vi "PJT_13.vi"() -> ()   [LabVIEW 2019]
panel:
  out "매칭된 숫자":dbl
  out "반복횟수":i32
  in  "입력숫자":dbl
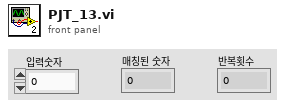
[diagram p1: front panel]
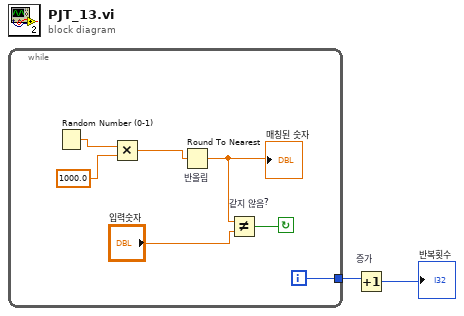
[diagram p0: block diagram]
diagram:
  n1 = while {
    tunnel: [w3] -> w2
    i -> [w3]
    stop <- w4 continue-if-true
    n2 = Random Number (0-1)() -> (number: 0 to 1=w8:dbl)
    n3 = Multiply(x=w8, y=1000.0) -> (x*y=w7:dbl)
    n4 = Round To Nearest "반올림"(number=w7) -> (nearest integer value=w6:dbl)
    "매칭된 숫자" <- w6
    n5 = Not Equal? "같지 않음?"(x=w6, y="입력숫자") -> (x != y?=w4:bool)
  }
  n6 = Increment "증가"(x=w2) -> (x+1=→"반복횟수":i32)
